vi "template-dense-cell.vi"(1 "x":T1) -> (0 "y":T1)   [LabVIEW 2020]
uses:
  <vilib>/Analysis/Matrix/Datatypes/RealMatrix.ctl
  <vilib>/Analysis/Matrix/Numeric/Conversions/Array To Matrix - RA2.vi
  <vilib>/Analysis/Matrix/Numeric/Multiply/Multiply - RM,RM.vi
  <vilib>/Analysis/Matrix/Numeric/Add/Add - RM,RM.vi
  <vilib>/Analysis/Matrix/NI_Matrix.lvlib
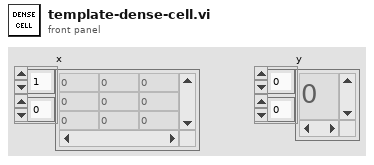
[diagram p1: front panel]
types:
  T1 = typedef "NI_Matrix.lvlib/RealMatrix.ctl" = dbl[][]
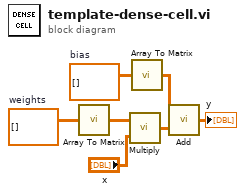
[diagram p0: block diagram]
diagram:
  w2 = dbl[][] []  # bias
  w6 = dbl[][] []  # weights
  n1 = call-poly <vilib>:"Array To Matrix.vi"("Real 2D Array"=w6) -> ("Real Matrix"=w5:T1)
  n2 = call-poly <vilib>:"Multiply.vi"("Real Matrix B"="x", "Real Matrix A"=w5) -> ("A * B"=w3:T1)
  n3 = call-poly <vilib>:"Array To Matrix.vi"("Real 2D Array"=w2) -> ("Real Matrix"=w1:T1)
  n4 = call-poly <vilib>:"Add.vi"("Real Matrix B"=w3, "Real Matrix A"=w1) -> ("A + B"=→"y":T1)
